vi "FPGA_I2C_Configure.vi"(8 "error in":errorcluster, 9 "Clock Rate (Hz)":dbl, 10 "Port":u8, 11 "FPGA VI Reference":T1) -> (0 "error out":errorcluster, 2 "Actual Rate (Hz)":dbl, 3 "FPGA VI Reference Out":T1)   [LabVIEW 2020, in "I2C Host API.lvlib"]
doc: "Sets the configuration options for an I2C port running on the FPGA. Specify port number and clock rate for the slave device."
uses:
  I2C Host API.lvlib
  RT/Controls/FPGA I2C_FPGA Ref.ctl
  FPGA/Controls/FPGA I2C_Cmd.ctl
  <vilib>/Utility/error.llb/Error Cluster From Error Code.vi
  <vilib>/rvi/errors/niLvFpgaAdjustHostInterfaceError.vi
  <vilib>/rvi/interface/nirviReadWriteControl/nirviReadWriteControl.xnode
  FPGA Bitfiles/I2CCommunication_FPGATarget2_I2CCommunication_VvdNkCkGvgg.lvbitx
  FPGA/FPGA-Main.vi
  NiFpgaLv.dll
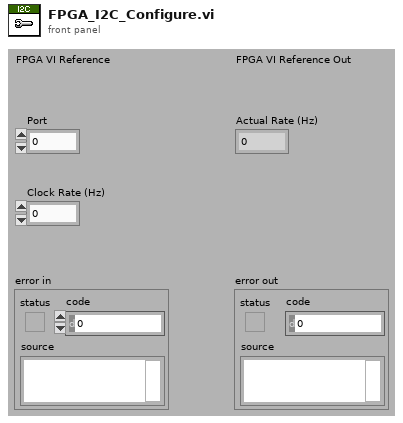
[diagram p1: front panel]
types:
  T1 = typedef "FPGA I2C_FPGA Ref.ctl" = refnum<k20>
  T2 = typedef "FPGA I2C_Cmd.ctl" = enum8{"Idle", "Write I2C", "Read I2C", "Write & Read I2C", "Configure"}
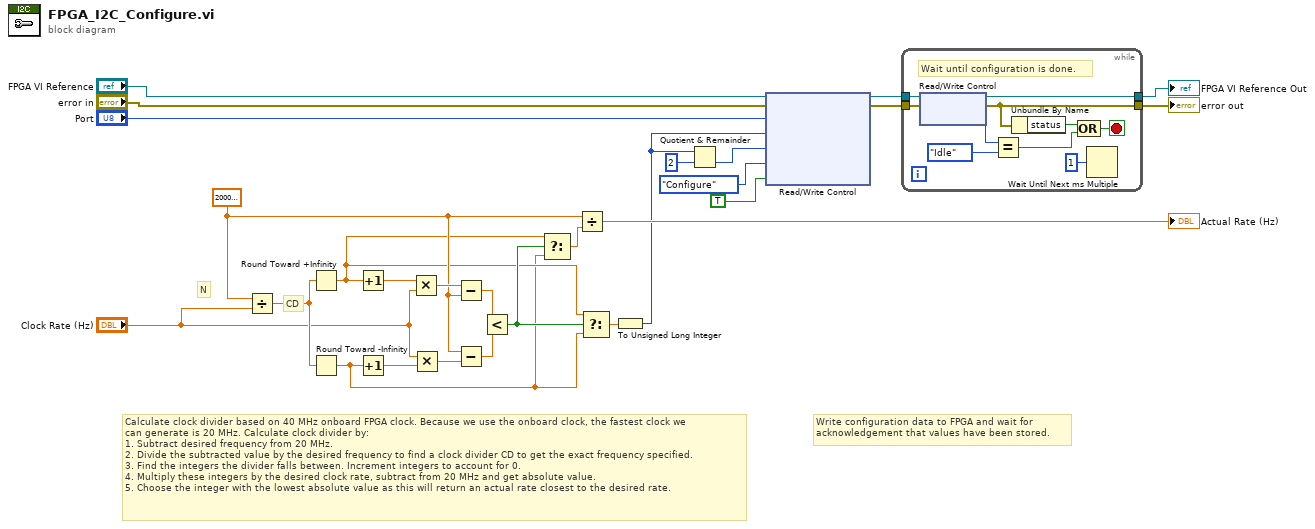
[diagram p0: block diagram]
diagram:
  w9 = 20000000.0 ("10M")
  # "Write configuration data to FPGA and wait for\nacknowledgement that values have been stored."
  # "Calculate clock divider based on 40 MHz onboard FPGA clock. Because we use the onboard clock, the fastest clock we\ncan generate is 20 MHz. Calculate clock divider by:\n1. Subtract desired frequency from 20 MHz.\n2. Divide the subtracted value by the desired frequency to find a clock divider CD to get the exact frequency specified.\n3. Find the integers the divider falls between. Increment integers to account for 0.\n4. Multiply these integers by the desired clock rate, subtract from 20 MHz and get absolute value.\n5. Choose the integer with the lowest absolute value as this will return an actual rate closest to the desired rate."
  # "CD"
  # "N"
  n1 = Divide(x=w9, y="Clock Rate (Hz)") -> (x/y=w20:dbl)
  n2 = Round Toward +Infinity(x=w20) -> (ceil(x): smallest int >= x=w8:dbl)
  n3 = Round Toward -Infinity(1:w20) -> (0:w7:dbl)
  n4 = Increment(x=w8) -> (x+1=w16:dbl)
  n5 = Increment(x=w7) -> (x+1=w17:dbl)
  n6 = Multiply(x=w16, y="Clock Rate (Hz)") -> (x*y=w24:dbl)
  n7 = Multiply(x="Clock Rate (Hz)", y=w17) -> (x*y=w23:dbl)
  n8 = Subtract(x=w24, y=w9) -> (x-y=w21:dbl)
  n9 = Subtract(x=w9, y=w23) -> (x-y=w22:dbl)
  n10 = Less?(x=w21, y=w22) -> (x < y?=w18:bool)
  n11 = Select(t=w8, s=w18, f=w7) -> (s? t:f=w19:dbl)
  n12 = Divide(x=w9, y=w19) -> (x/y=→"Actual Rate (Hz)":dbl)
  n13 = Select(t=w8, s=w18, f=w7) -> (s? t:f=w14:dbl)
  n14 = To Unsigned Long Integer(number=w14) -> (unsigned 32bit integer=w6:u32)
  n15 = Quotient & Remainder(x=w6, y=u32 2) -> (floor(x/y)=w4:u32)  [unwired: 1 out]
  n16 = xnode "Read/Write Control"("FPGA VI Reference In"="FPGA VI Reference", "error in"="error in", "I2C_Port"="Port", "I2C_Wait Time"=w6, "I2C_Wait Time/2"=w4, "I2C_Cmd"=FPGA_I2C_Cmd."Configure", "I2C_Start"=TRUE) -> ("FPGA VI Reference Out"=w13:T1, "error out"=w11:errorcluster)
  n17 = while {
    tunnel: w13 -> [w37]
    tunnel: [w36] -> w12
    tunnel: w11 -> [w35]
    tunnel: [w34] -> w10
    stop <- w31 stop-if-true
    # "Wait until configuration is done."
    n18 = xnode "Read/Write Control"("FPGA VI Reference In"=w37, "error in"=w35) -> ("FPGA VI Reference Out"=w36:T1, "error out"=w34:errorcluster, "I2C_Cmd"=w28:T2)
    n19 = Equal?(x=w28, y=FPGA_I2C_Cmd."Idle" ("I2C_Cmd")) -> (x = y?=w32:bool)
    n20 = Unbundle By Name(w34) -> ("status"=w33:bool)
    n21 = Compound Arithmetic op=OR(w33, w32) -> (w31:bool)
    n22 = Wait Until Next ms Multiple(millisecond multiple=u32 1) -> ()  [unwired: 1 out]
  }
  "error out" <- w10
  "FPGA VI Reference Out" <- w12
